vi "ShortestDistanceBetweenRegimes.vi"(10 "Regime 2":T1, 11 "Regime 1":T1) -> (3 "Distance between the two regimes":i32)   [LabVIEW 2013]
doc: "This takes in two sailing regimes and returns the minimum absolute distance between those two regimes. If the regimes are adjacent, for example, this VI will return '1' for 'Distance between the two regimes'.\n\nIt also indicates by -1, 0, or 1 which direction Regime 2 is from Regime 1. For example, if Current Regime is passed into Regime 1 and Desired Regime is passed into Regime 2, the 'Direction to Regime 2' will return the direction to the desired heading, whether that be in the positive (1) or negative (-1) direction. 0 means you are already there.\n\nEric Schneider, Feb. 2014"
uses:
  Data/TypeDefs/Sailing Regimes.ctl
panel:
  out "Direction to Regime 2":i32
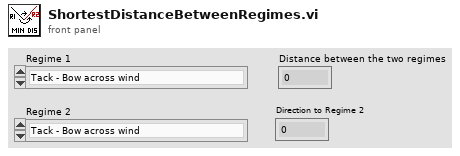
[diagram p1: front panel]
types:
  T1 = typedef "Sailing Regimes.ctl" = enum16{"Tack - Bow across wind", "Upwind - Starboard Tack", "Turn between Upwind/Reach - Starboard Tack", "Reach - Starboard Tack", "Turn between Reach/Run - Starboard Tack", "Run - Starboard Tack", "Jibe - Stern across wind", "Run - Port Tack", "Turn between Reach/Run - Port Tack", "Reach - Port Tack", "Turn between Upwind/Reach - Port Tack", "Upwind - Port Tack"}
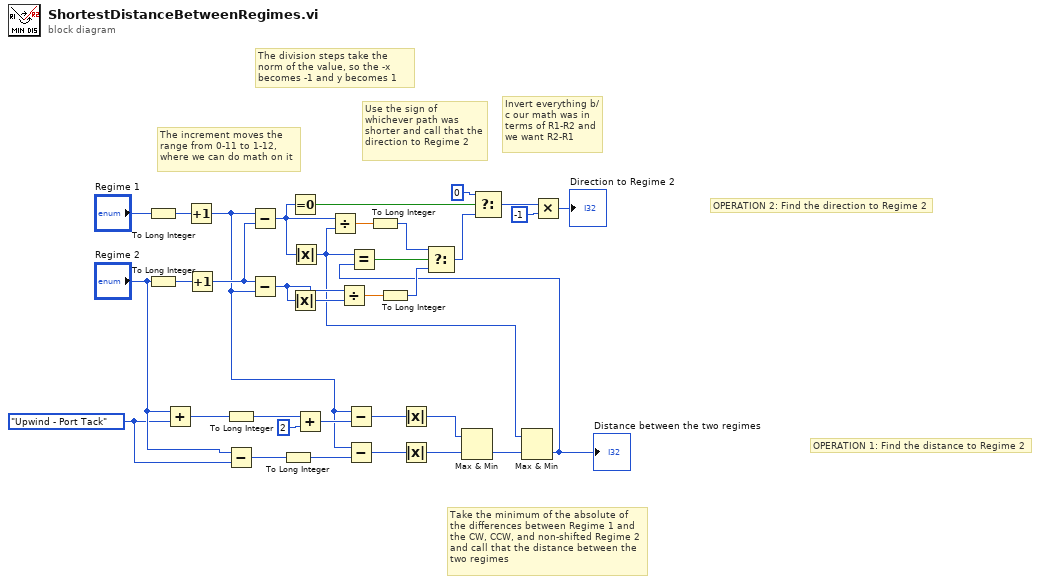
[diagram p0: block diagram]
diagram:
  w2 = Sailing_Regimes."Upwind - Port Tack" ("y")
  # "Invert everything b/c our math was in terms of R1-R2 and we want R2-R1"
  # "OPERATION 1: Find the distance to Regime 2"
  # "OPERATION 2: Find the direction to Regime 2"
  # "The increment moves the range from 0-11 to 1-12, where we can do math on it"
  # "Take the minimum of the absolute of the differences between Regime 1 and the CW, CCW, and non-shifted Regime 2 and call that the distance between the two regimes"
  # "Use the sign of whichever path was shorter and call that the direction to Regime 2"
  # "The division steps take the norm of the value, so the -x becomes -1 and y becomes 1"
  n1 = To Long Integer(number="Regime 1") -> (32bit integer=w15:i32)
  n2 = To Long Integer(number="Regime 2") -> (32bit integer=w14:i32)
  n3 = Add(x="Regime 2", y=w2) -> (x+y=w33:u16)
  n4 = Increment(x=w15) -> (x+1=w1:i32)
  n5 = Increment(x=w14) -> (x+1=w13:i32)
  n6 = To Long Integer(number=w33) -> (32bit integer=w12:i32)
  n7 = Subtract(x="Regime 2", y=w2) -> (x-y=w9:u16)
  n8 = Subtract(x=w1, y=w13) -> (x-y=w30:i32)
  n9 = Subtract(x=w13, y=w1) -> (x-y=w23:i32)
  n10 = To Long Integer(number=w9) -> (32bit integer=w7:i32)
  n11 = Equal To 0?(x=w30) -> (x = 0?=w32:bool)
  n12 = Absolute Value(x=w23) -> (abs(x)=w22:i32)
  n13 = Absolute Value(x=w30) -> (abs(x)=w21:i32)
  n14 = Add(x=w12, y=2) -> (x+y=w10:i32)
  n15 = Divide(x=w30, y=w21) -> (x/y=w29:dbl)
  n16 = Divide(x=w23, y=w22) -> (x/y=w26:dbl)
  n17 = Subtract(x=w1, y=w10) -> (x-y=w24:i32)
  n18 = Subtract(x=w1, y=w7) -> (x-y=w6:i32)
  n19 = To Long Integer(number=w29) -> (32bit integer=w28:i32)
  n20 = To Long Integer(number=w26) -> (32bit integer=w25:i32)
  n21 = Absolute Value(x=w24) -> (abs(x)=w4:i32)
  n22 = Absolute Value(x=w6) -> (abs(x)=w5:i32)
  n23 = Max & Min(x=w4, y=w5) -> (min(x,y)=w3:i32)  [unwired: 1 out]
  n24 = Max & Min(x=w21, y=w3) -> (min(x,y)=w20:i32)  [unwired: 1 out]
  "Distance between the two regimes" <- w20
  n25 = Equal?(x=w21, y=w20) -> (x = y?=w19:bool)
  n26 = Select(t=w28, s=w19, f=w25) -> (s? t:f=w27:i32)
  n27 = Select(t=0, s=w32, f=w27) -> (s? t:f=w18:i32)
  n28 = Multiply(x=w18, y=-1) -> (x*y=→"Direction to Regime 2":i32)
